vi "CalcRotationAngles.vi"(8 "ZAxis":dbl, 10 "YAxis":dbl, 11 "XAxis":dbl) -> (2 "Speeds":dbl[](array[numeric]), 3 "Angles":dbl[](array[numeric]))   [LabVIEW 2018]
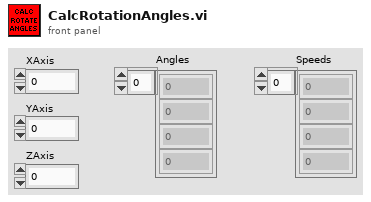
[diagram p1: front panel]
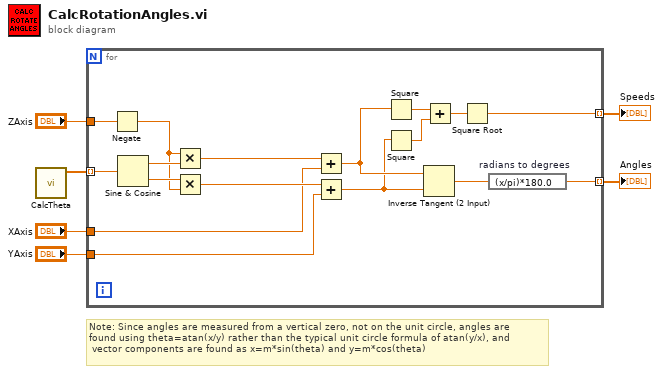
[diagram p0: block diagram]
diagram:
  # "Note: Since angles are measured from a vertical zero, not on the unit circle, angles are\nfound using theta=atan(x/y) rather than the typical unit circle formula of atan(y/x), and\n vector components are found as x=m*sin(theta) and y=m*cos(theta)"
  n1 = call "CalcTheta.vi"() -> ("ThetaValues"=w2:dbl[])  [unwired: 11 in]
  n2 = for {
    tunnel: w2 -> [w21] mode=indexing
    tunnel: "ZAxis" -> [w20]
    tunnel: "YAxis" -> [w7]
    tunnel: "XAxis" -> [w8]
    tunnel: [w23] -> w5 mode=indexing
    tunnel: [w22] -> w6 mode=indexing
    n3 = Negate(x=w20) -> (-x=w12:dbl)
    n4 = Sine & Cosine(0:w21) -> (1:w15:dbl, 2:w14:dbl)
    n5 = Multiply(x=w12, y=w15) -> (x*y=w13:dbl)
    n6 = Multiply(x=w14, y=w12) -> (x*y=w9:dbl)
    n7 = Add(x=w13, y=w8) -> (x+y=w11:dbl)
    n8 = Add(x=w9, y=w7) -> (x+y=w10:dbl)
    n9 = Square(x=w11) -> (x^2=w18:dbl)
    n10 = Square(x=w10) -> (x^2=w17:dbl)
    n11 = Inverse Tangent (2 Input)(1:w10, 2:w11) -> (0:w19:dbl)
    n12 = Add(x=w18, y=w17) -> (x+y=w16:dbl)
    n13 = Square Root(x=w16) -> (sqrt(x)=w22:dbl)
    n14 = expression code="(x/pi)*180.0" "radians to degrees"(w19) -> (w23:dbl)
  }
  "Angles" <- w5
  "Speeds" <- w6
